vi "mixture_enthalpy_quality.vi"(4 "Vapor Inlet Pressure [Pa]":dbl, 5 "Separator Temp [C]":dbl, 6 "Liquid Inlet Temp [C]":dbl, 7 "Vapor Flow Rate [g/s]":dbl, 8 "Liquid Flow Rate [g/s]":dbl) -> (0 "Quality [-]":dbl, 1 "mixture enthalpy":dbl, 2 "h_v_corr":dbl, 3 "h_l_corr":dbl)   [LabVIEW 2017]
uses:
  <vilib>/express/express arith-compare/Formula/XNode/ExpressFormulaBlockNode.xnode
  Sensor Translation/sensor_translation.lvlib
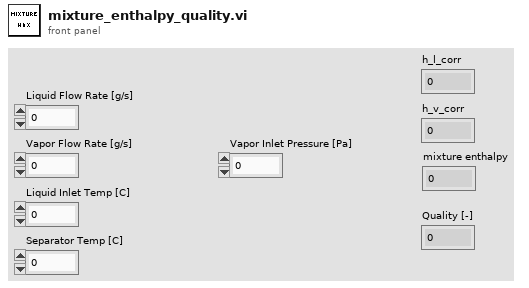
[diagram p1: front panel]
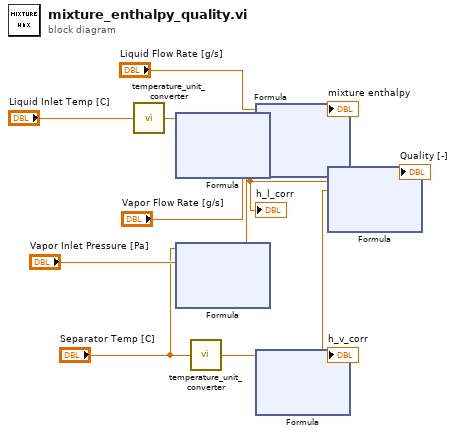
[diagram p0: block diagram]
diagram:
  n1 = call "temperature_unit_converter.vi"("Input"="Liquid Inlet Temp [C]") -> ("Output"=w1:dbl)  [unwired: 2 in]
  n2 = xnode "Formula"("T"=w1) -> ("Result"=w6:dbl)  [unwired: 1 in, 1 out]
  "h_l_corr" <- w6
  n3 = xnode "Formula"("T_v"="Separator Temp [C]", "P_v"="Vapor Inlet Pressure [Pa]") -> ("Result"=w10:dbl)  [unwired: 1 in, 1 out]
  n4 = call "temperature_unit_converter.vi"("Input"="Separator Temp [C]") -> ("Output"=w3:dbl)  [unwired: 2 in]
  n5 = xnode "Formula"("m_dot_l"="Liquid Flow Rate [g/s]", "h_l"=w6, "m_dot_v"="Vapor Flow Rate [g/s]", "h_v"=w10) -> ("Result"=w8:dbl)  [unwired: 1 in, 1 out]
  "mixture enthalpy" <- w8
  n6 = xnode "Formula"("T"=w3) -> ("Result"=w7:dbl)  [unwired: 1 in, 1 out]
  "h_v_corr" <- w7
  n7 = xnode "Formula"("h_mix"=w8, "h_l"=w6, "h_v"=w7) -> ("Result"=→"Quality [-]":dbl)  [unwired: 1 in, 1 out]
